vi "CalcCurrentThreshold.vi"(7 "Target Decimal Output":u8=1, 9 "Current Threshold":dbl=1000.0 format="%#_13g", 10 "Current of Output Pins":dbl[](array[numeric])) -> (0 "Current Threshold":dbl=1000.0 format="%#_13g", 3 "Target binary output":bool[](array[boolean]))   [LabVIEW 2018]
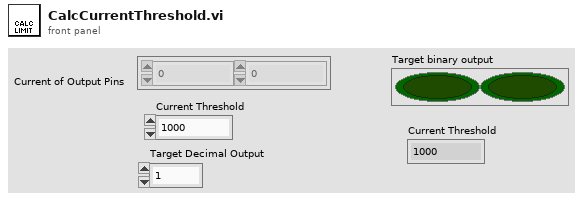
[diagram p1: front panel]
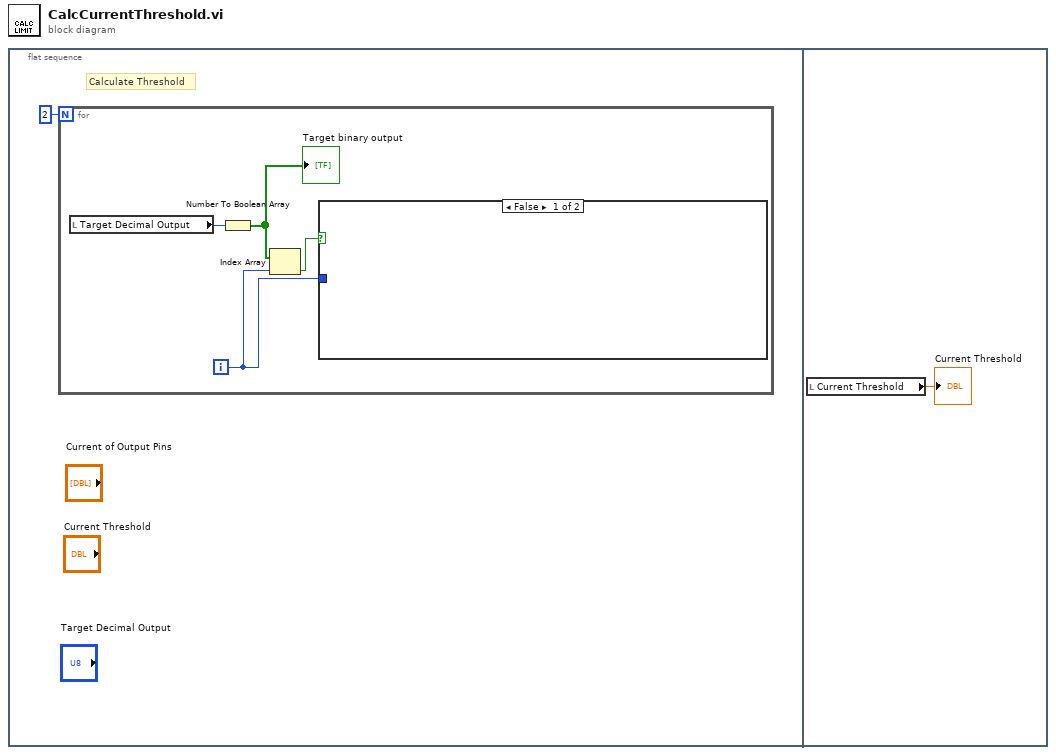
[diagram p0: block diagram]
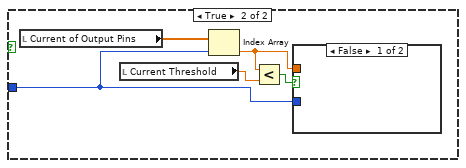
[diagram p2: hidden frame]
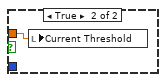
[diagram p3: hidden frame]
diagram:
  n1 = flat-sequence {
    frame #0 {
      # "Calculate Threshold"
      n2 = for {
        N: 2 -> [_]
        i -> [w3]
        n3 = local read "Target Decimal Output"() -> (w5:u8)
        n4 = Number To Boolean Array(number=w5) -> (Boolean array=w2:bool[])
        "Target binary output" <- w2
        n5 = Index Array(array=w2, index=w3) -> (element=w4:bool)
        n6 = case shown="False" w4 {
          tunnel: w3 -> [_ w10]
          frame False {
          }
          frame True {
            n7 = local read "Current of Output Pins"() -> (w8:dbl[])
            n8 = local read "Current Threshold"() -> (w6:dbl)
            n9 = Index Array(array=w8, index=w10) -> (element=w7:dbl)
            n10 = Less?(x=w7, y=w6) -> (x < y?=w9:bool)
            n11 = case shown="False" w9 {
              tunnel: w10 -> [_ _]
              tunnel: w7 -> [_ w11]
              frame False {
              }
              frame True {
                n12 = local write "Current Threshold"(w11) -> ()
              }
            }
          }
        }
      }
    }
    frame #1 {
      n13 = local read "Current Threshold"() -> (→"Current Threshold":dbl)
    }
  }
